vi "Example8.vi"() -> ()   [LabVIEW 2019]
panel:
  out "I":dbl
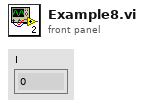
[diagram p1: front panel]
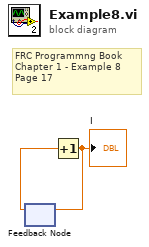
[diagram p0: block diagram]
diagram:
  # "FRC Programmng Book\nChapter 1 - Example 8\nPage 17"
  n1 = feedback #1() -> (w1:dbl)  [unwired: 1 in]
  n2 = Increment(x=w1) -> (x+1=w2:dbl)
  "I" <- w2
  n3 = feedback-in #1(w2) -> ()
